vi "Init PTC10.vi"(8 "error in (no error)":errorcluster, 11 "PTC10":T1={"serial settings"={"port"="Stanford_PTC10", "baud rate"=9600}, "PTC10 Info"={"Manufacturer"="", "Instrument"="", "Serial Number"="", "Firmware"=""}, "VISA resource name"="", "pwmloop"="define pwmloop(#t=0 while (1) {waitforsample if(#pwm=0){relays=0}else{if(#t<#pwm) {relays=1}else{relays=3}}#t+=1 if  (#t>99){#t=0} pause 0.2 s})", "onecycle"="define onecycle (pwm=100 run pwmloop 5A.PID.Setpoint=-130.0 5A.PID.input=3C while(#3C>-129.0){pause 0.2 s}pwm=-130 pause 10 min pwm=0  5A.PID.SetPoint=50.0 while(#3C<49.0){pause 0.2 s} pause 10 min kill pwmloop)", "control"="define control (#count=1 while (#count>=0) {onecycle pause 1 s #count-=1})", "HeatDrive"="define Failsafe (while(1) {if (#Check <-20){relays=0 outputEnable Off}else{if(#Check>20){relays=0 outputEnable Off}} pause 1 s})", "ToAmbient"="define ToAmbient(if(#3C>25.0){pwm=100 run pwmloop while(#3C>#25.0){pause 0.5 s} pwm=0 kill pwmloop}else{#5A.PID.setpoint=20.0 while(#3C<15.0){pause 0.5 s} outputenable off})", "StartupCode"="system.display.Monitors Show", "LogChannels"=[], "Heater O/P Channel"="", " Control Input"="", "TAmbient"=20.0, "AmbientTolerance"=5.0, "TestCycleParameters"={"TAmb"=20.0, "HeaterTestTemp"=-80.0, "HeaterTestDwell(min)"=30, "HeaterTestDuration"=15, "MinOpTemp"=-50.0, "MinOpDwell(min)"=30, "TestHeatingRate (deg/min)"=0.4, "SurviveCycleParameters"={"MinSurviveTemp"=-131.5, "MinSurvive Dwell(min)"=10, "MaxSurviveTemp"=50.0, "MaxSurviveDwell(min)"=30, "ControlInput"=2, "ColdStandOff"=4.0, "HotStandoff"=5.0, "SteadyPWM"=20, "MaxCoolingRate (deg/min)"=3.75, "MaxHeatingRate (deg/min)"=2.5}, "CycleType"=0, "MaxOpTemp"=-50.0, "MaxOpDwell(min)"=30}, "PID Params"={"P"=1.14, "I"=0.012, "D"=21.68, "Set"=0.0}} {"PID Params"."D" min=0.0; "PID Params"."I" min=0.0; "PID Params"."P" min=0.0; "TestCycleParameters"."CycleType" items=["Survival", "Operational"]; "TestCycleParameters"."SurviveCycleParameters"."SteadyPWM" min=0 max=100 step=1; "TestCycleParameters"."SurviveCycleParameters"."ControlInput" items=["3A", "3B", "3C", "3D", "4A", "4B", "4C", "4D"]; "serial settings"."baud rate" items=["9600"=9600, "19200"=19200, "38400"=38400, "57600"=57600, "115200"=115200]}) -> (0 "error out":errorcluster, 3 "PTC10 Out":T1={"serial settings"={"port"="", "baud rate"=115200}, "PTC10 Info"={"Manufacturer"="", "Instrument"="", "Serial Number"="", "Firmware"=""}, "VISA resource name"="", "pwmloop"="define coldloop(while (1) {if (#3C > -130.0) {relays&=13} if (#3C < -130.0){relays|=2} pause 0.1 s })", "onecycle"="define onecycle (relays=1 while(#3C >-129.0){pause 0.1 s} relays|=2 pause 30 s run\"coldloop\" pause 10 min kill\"coldloop\" relays=4 while(#3C<49.0){pause 0.1 s} pause 10 s run\"hotloop\" pause 10 min kill\"hotloop\" relays=0)", "control"="define control (#count=1 while (#count>0) {onecycle pause 1 s #count-=1})", "HeatDrive"="define coldloop(while (1) {if (#3C > -130.0) {relays&=13} if (#3C < -130.0){relays|=2} pause 0.1 s })", "ToAmbient"="define ToAmbient(if(#3C>25.0){pwm=100 run pwmloop while(#3C>#25.0){pause 0.5 s} pwm=0 kill pwmloop}else{#5A.PID.setpoint=20.0 while(#3C<15.0){pause 0.5 s} outputenable off})", "StartupCode"="system.display.Monitors Show", "LogChannels"=[], "Heater O/P Channel"="", " Control Input"="", "TAmbient"=20.0, "AmbientTolerance"=5.0, "TestCycleParameters"={"TAmb"=20.0, "HeaterTestTemp"=20.0, "HeaterTestDwell(min)"=1, "HeaterTestDuration"=1, "MinOpTemp"=-131.5, "MinOpDwell(min)"=30, "TestHeatingRate (deg/min)"=0.4, "SurviveCycleParameters"={"MinSurviveTemp"=-131.5, "MinSurvive Dwell(min)"=10, "MaxSurviveTemp"=50.0, "MaxSurviveDwell(min)"=30, "ControlInput"=2, "ColdStandOff"=4.0, "HotStandoff"=5.0, "SteadyPWM"=20, "MaxCoolingRate (deg/min)"=3.75, "MaxHeatingRate (deg/min)"=2.5}, "CycleType"=0, "MaxOpTemp"=-50.0, "MaxOpDwell(min)"=30}, "PID Params"={"P"=1.14, "I"=0.012, "D"=21.68, "Set"=0.0}} {"PID Params"."D" min=0.0; "PID Params"."I" min=0.0; "PID Params"."P" min=0.0; "TestCycleParameters"."CycleType" items=["Survival", "Operational"]; "TestCycleParameters"."SurviveCycleParameters"."SteadyPWM" min=0 max=100 step=1; "TestCycleParameters"."SurviveCycleParameters"."ControlInput" items=["3A", "3B", "3C", "3D", "4A", "4B", "4C", "4D"]; "serial settings"."baud rate" items=["9600"=9600, "19200"=19200, "38400"=38400, "57600"=57600, "115200"=115200]})   [LabVIEW 2024]
uses:
  controls/SRS PTC10.ctl
  controls/TestCycleParams.ctl
  controls/SurviveCycleParams.ctl
  controls/ControlInput.ctl
  controls/PID Params.ctl
  <vilib>/Instr/_visa.llb/VISA Flush IO Buffer Mask.ctl
  <vilib>/Utility/error.llb/Trim Whitespace One-Sided.vi
  <instrlib>/Stanford PTC10/SRS PTC10.lvlib
panel:
  out "General Settings:Timeout Value":u32
  out "Channels":string
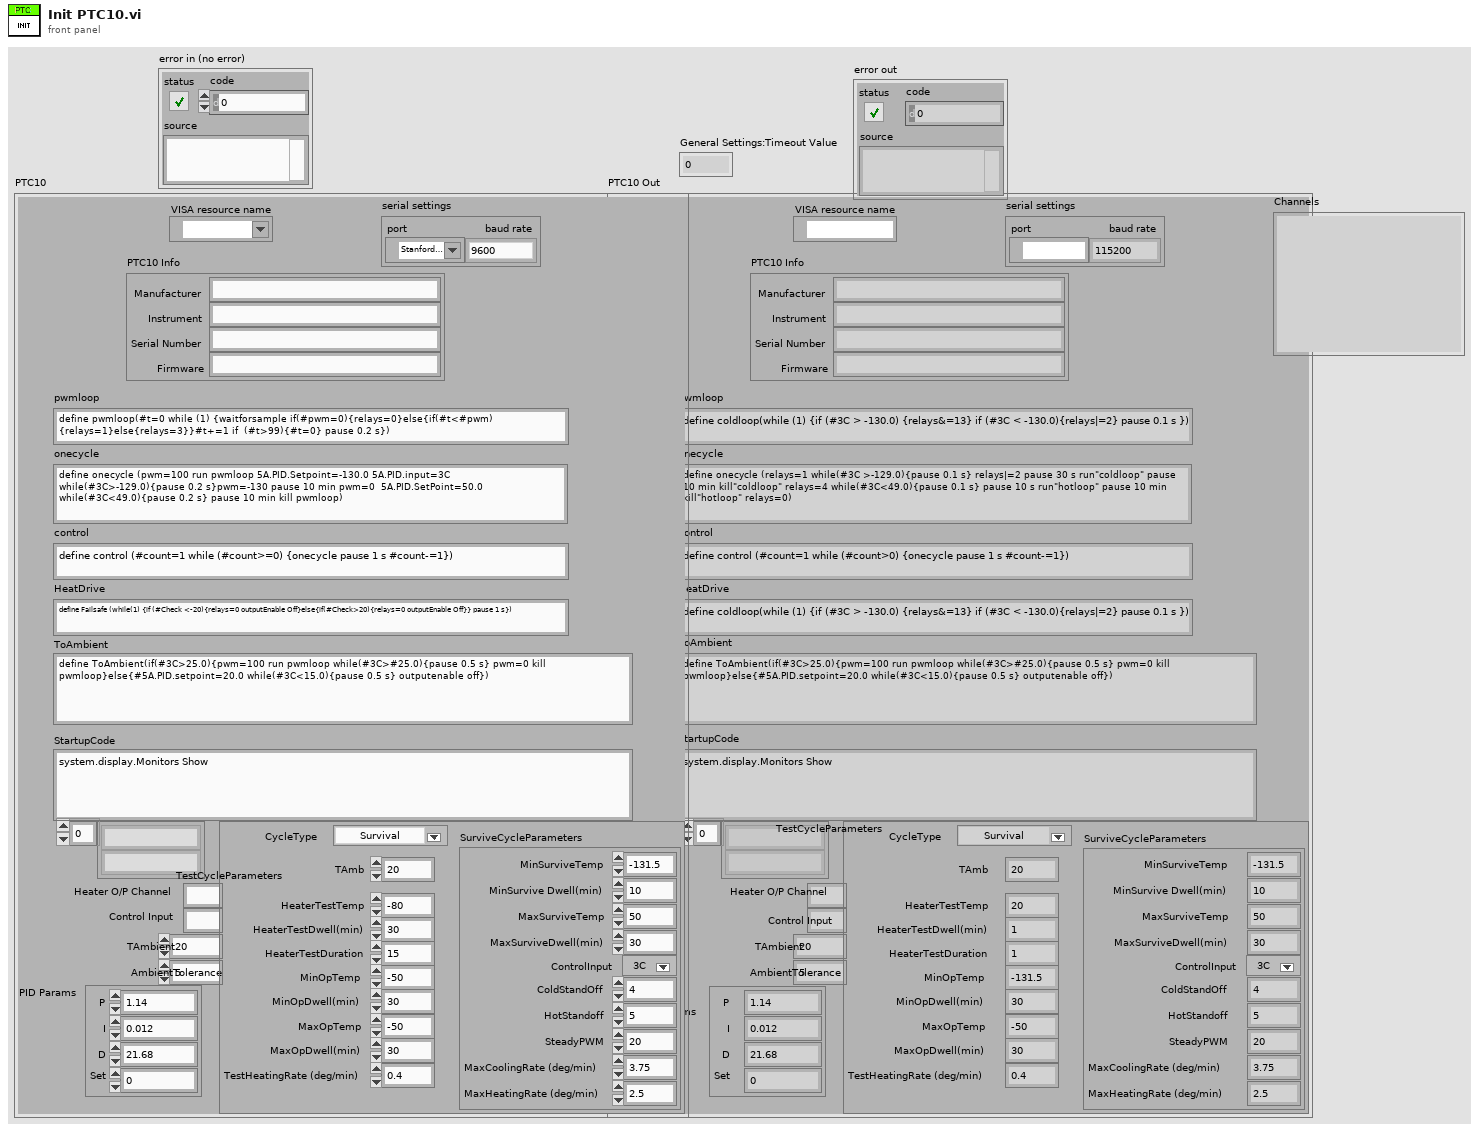
[diagram p1: front panel]
types:
  T1 = typedef "SRS PTC10.ctl" = cluster{"serial settings":cluster{"port":refnum<visa-resource-name>, "baud rate":u32}, "PTC10 Info":cluster{"Manufacturer":string, "Instrument":string, "Serial Number":string, "Firmware":string}, "VISA resource name":refnum<visa-resource-name>, "pwmloop":string, "onecycle":string, "control":string, "HeatDrive":string, "ToAmbient":string, "StartupCode":string, "LogChannels":string[], "Heater O/P Channel":string, " Control Input":string, "TAmbient":dbl, "AmbientTolerance":dbl, "TestCycleParameters":T2, "PID Params":T5}
  T2 = typedef "TestCycleParams.ctl" = cluster{"TAmb":dbl, "HeaterTestTemp":dbl, "HeaterTestDwell(min)":i32, "HeaterTestDuration":i32, "MinOpTemp":dbl, "MinOpDwell(min)":i32, "TestHeatingRate (deg/min)":dbl, "SurviveCycleParameters":T3, "CycleType":u16, "MaxOpTemp":dbl, "MaxOpDwell(min)":i32}
  T3 = typedef "SurviveCycleParams.ctl" = cluster{"MinSurviveTemp":dbl, "MinSurvive Dwell(min)":i32, "MaxSurviveTemp":dbl, "MaxSurviveDwell(min)":i32, "ControlInput":T4, "ColdStandOff":dbl, "HotStandoff":dbl, "SteadyPWM":i32, "MaxCoolingRate (deg/min)":dbl, "MaxHeatingRate (deg/min)":dbl}
  T4 = typedef "ControlInput.ctl" = u16
  T5 = typedef "PID Params.ctl" = cluster{"P":dbl, "I":dbl, "D":dbl, "Set":dbl}
  T6 = typedef "VISA Flush IO Buffer Mask.ctl" = u16
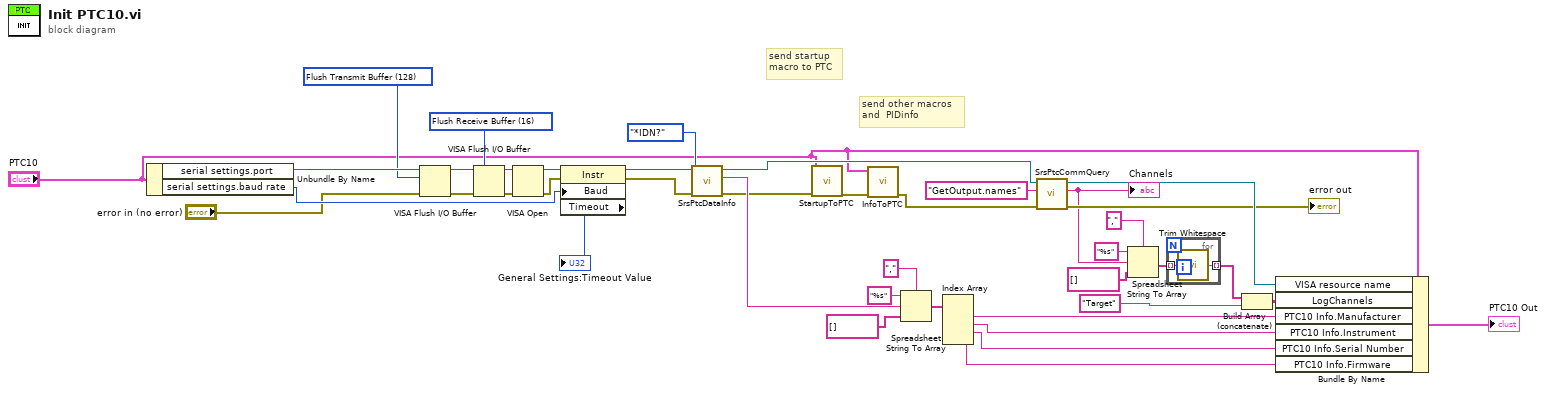
[diagram p0: block diagram]
diagram:
  w16 = T6 128 items=["Flush Receive Buffer"=16, "Write Transmit Buffer to Device"=32, "Flush Receive Buffer (No I/O)"=64, "Flush Transmit Buffer"=128] ("Mask")
  w21 = T6 16 items=["Flush Receive Buffer"=16, "Write Transmit Buffer to Device"=32, "Flush Receive Buffer (No I/O)"=64, "Flush Transmit Buffer"=128] ("Mask")
  # "send other macros \nand  PIDinfo"
  # "send startup \nmacro to PTC"
  n1 = Unbundle By Name("PTC10") -> ("serial settings.port"=w17:refnum<visa-resource-name>, "serial settings.baud rate"=w39:u32)
  n2 = VISA Flush I/O Buffer(VISA resource name=w17, mask (16)=w16, error in (no error)="error in (no error)") -> (VISA resource name out=w20:refnum<visa-resource-name>, error out=w19:errorcluster)
  n3 = VISA Flush I/O Buffer(VISA resource name=w20, mask (16)=w21, error in (no error)=w19) -> (VISA resource name out=w23:refnum<visa-resource-name>, error out=w22:errorcluster)
  n4 = VISA Open(error in (no error)=w22, VISA resource name=w23) -> (VISA resource name=w40:refnum<visa-resource-name>, error out=w36:errorcluster)  [unwired: 3 in]
  n5 = property class="Instr"(reference=w40, error in=w36, "Baud"=w39) -> (reference out=w38:refnum<visa-resource-name>, error out=w37:errorcluster, "Timeout"=→"General Settings:Timeout Value":u32)
  n6 = call <instrlib>:"SrsPtcDataInfo.vi"("error in"=w37, "Type of Info"=enum8{"*IDN?", "description?"}."*IDN?", "SRS PTC10 VISA in"=w38) -> ("error out"=w10:errorcluster, "Output"=w32:string, "SRS PTC10 VISA out"=w9:refnum<visa-resource-name>)  [unwired: 6 in]
  n7 = call "StartupToPTC.vi"("error in (no error)"=w10, "PTC10 In"="PTC10") -> ("error out"=w6:errorcluster)  [unwired: 9 in]
  n8 = call "InfoToPTC.vi"("error in (no error)"=w6, "PTC10"="PTC10") -> ("error out"=w5:errorcluster)  [unwired: 9 in]
  n9 = Spreadsheet String To Array(delimiter (Tab)=",", format string="%s", spreadsheet string=w32, array type (2D Dbl)=string[] []) -> (array=w31:string[])
  n10 = Index Array(array=w31) -> (element #1=w11:string, element #2=w30:string, element #3=w29:string, element #4=w28:string)  [unwired: 4 in]
  n11 = call <instrlib>:"SrsPtcCommQuery.vi"("error in"=w5, "Command"="GetOutput.names", "SRS PTC10 VISA in"=w9) -> ("error out"=→"error out":errorcluster, "Output"=w12:string, "SRS PTC10 VISA out"=w27:refnum<visa-resource-name>)  [unwired: 3 in, 3 out]
  "Channels" <- w12
  n12 = Spreadsheet String To Array(delimiter (Tab)=",", format string="%s", spreadsheet string=w12, array type (2D Dbl)=string[] []) -> (array=w2:string[])
  n13 = for {
    tunnel: w2 -> [w43] mode=indexing
    tunnel: [w42] -> w1 mode=indexing
    n14 = call <vilib>:"Trim Whitespace.vi"("string"=w43) -> ("trimmed string"=w42:string)  [unwired: 1 in]
  }
  n15 = Build Array (concatenate)(w1, "Target" ("format string")) -> (w8:string[])
  n16 = Bundle By Name(cluster="PTC10", "VISA resource name"=w27, "LogChannels"=w8, "PTC10 Info.Manufacturer"=w11, "PTC10 Info.Instrument"=w30, "PTC10 Info.Serial Number"=w29, "PTC10 Info.Firmware"=w28) -> (→"PTC10 Out":T1)
